vi "test_DMA Channels Input.vi"(8 "error in (no error)":errorcluster, 11 "TestCase in":refnum<class "DMA Channel Testing.lvclass">) -> (0 "error out":errorcluster, 3 "TestCase out":refnum<class "DMA Channel Testing.lvclass">)   [LabVIEW 2019, in "DMA Channel Testing.lvclass"]
uses:
  DMA Channel Testing.lvclass
  Addon/Addon Shared/Types/DMA Settings.ctl
  Addon/Addon Shared/Types/Delacing Scheme.ctl
  Addon/Addon Shared/Types/DMA Acquisition Mode.ctl
  DMA Channel Testing.lvclass/DMA Channel Testing.ctl
  Addon/Addon Shared/SubVIs/Constants.vi
  <vilib>/NI/NI VeriStand Advanced SysDef API/_SubVIs/SysDef.Search.GUID.vi
  <vilib>/NI/NI VeriStand Advanced SysDef API/_SubVIs/SysDef.Search.GUIDs.vi
  <vilib>/addons/_JKI Toolkits/VI Tester/TestCase.llb/TestCase.lvclass
  Addon/Addon System Explorer/FPGA Addon System Explorer.lvlib
  Addon/Addon Shared/FPGA Addon Shared.lvlib
  <vilib>/NI/NI VeriStand Advanced SysDef API/SysDef API/Advanced System Definition.lvlib
  C:/Program Files (x86)/National Instruments/LabVIEW 2019/vi.lib/addons/_JKI Toolkits/VI Tester/TestCase.llb/TestCase.lvclass
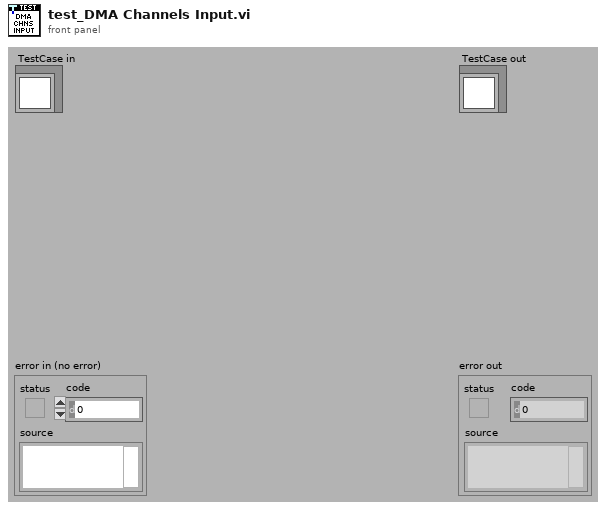
[diagram p1: front panel]
types:
  T1 = typedef "FPGA Addon Shared.lvlib/DMA Settings.ctl" = cluster{"Number of Channels":u8, "Delacing Scheme":T2, "Update Rate":u32, "dt":dbl, "Mode":T3, "Number of Samples":u32, "DMA Host Buffer":u32}
  T2 = typedef "FPGA Addon Shared.lvlib/Delacing Scheme.ctl" = enum8{"Interleaved", "Bitpacked"}
  T3 = typedef "FPGA Addon Shared.lvlib/DMA Acquisition Mode.ctl" = enum8{"Continuous", "Triggered Finite"}
  T4 = typedef "Advanced System Definition.lvlib/TreeItem.Info.ctl" = cluster{"Name":string, "Description":string, "GUID":string, "Is Channel":bool, "Channel":T5, "Is Waveform":bool, "Waveform":T7}
  T5 = typedef "Custom Device API.lvlib/Custom Device Channel.ctl" = cluster{"Type":T6, "Units":string, "Default Value":dbl, "Faultable":bool, "Scalable":bool}
  T6 = typedef "Custom Device API.lvlib/Custom Device Channel Type.ctl" = enum16{"Input", "Output"}
  T7 = typedef "Custom Device API.lvlib/Custom Device Waveform.ctl" = cluster{"Data Type":T8, "Units":string}
  T8 = typedef "Custom Device API.lvlib/Custom Device Waveform DataType.ctl" = enum16{"Double", "Complex Double"}
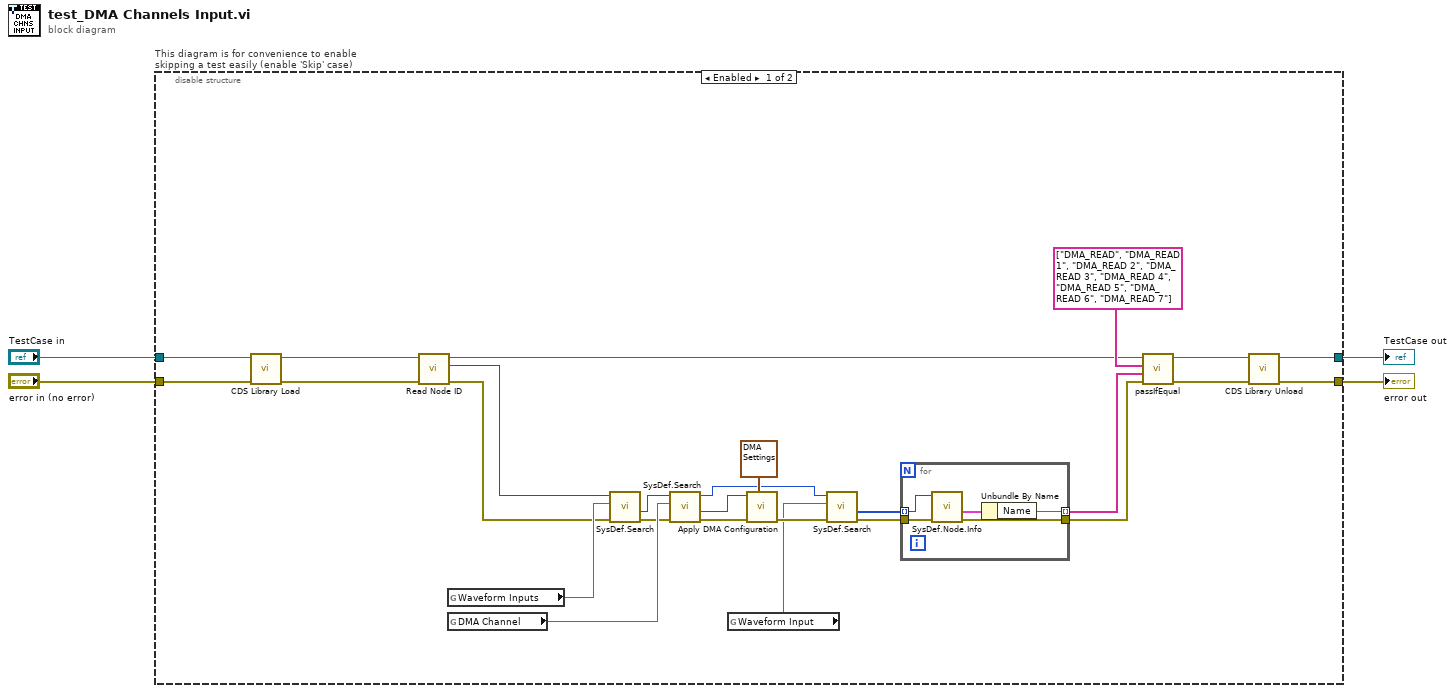
[diagram p0: block diagram]
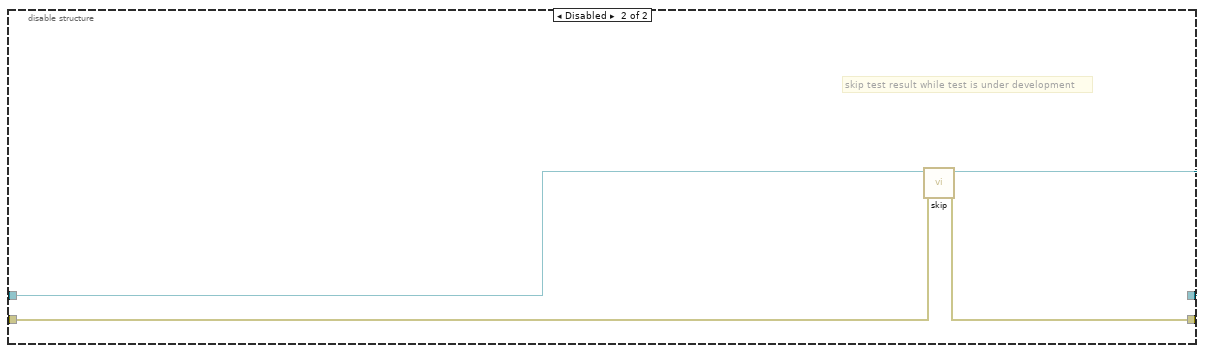
[diagram p2: hidden frame]
diagram:
  n1 = disable-structure "This diagram is for convenience to enable skipping a test easily (enable 'Skip' case)" shown="Enabled" {
    disable-tunnel: "TestCase in" -> [w11 w39]
    disable-tunnel: [w5 w37] -> w1
    disable-tunnel: [w6 w38] -> w3
    disable-tunnel: "error in (no error)" -> [w12 w36]
    frame Enabled {
      n2 = call "CDS Library Load.vi"("error in (no error)"=w12, "DMA Channel Testing in"=w11) -> ("error out"=w9:errorcluster, "DMA Channel Testing out"=w10:refnum<class "DMA Channel Testing.lvclass">)  [unwired: 8 in]
      n3 = call "Read Node ID.vi"("error in (no error)"=w9, "DMA Channel Testing in"=w10) -> ("error out"=w15:errorcluster, "Node ID"=w14:u64, "DMA Channel Testing out"=w13:refnum<class "DMA Channel Testing.lvclass">)  [unwired: 7 in]
      n4 = global read "Constants.vi" "Waveform Inputs"() -> (w28:string)
      n5 = global read "Constants.vi" "DMA Channel"() -> (w27:string)
      n6 = call-poly <vilib>:"SysDef.Search.vi"("error in (no error)"=w15, "GUID"=w28, "nodeID"=w14) -> ("error out"=w25:errorcluster, "Value out"=w26:u64)  [unwired: 5 in, 2 out]
      n7 = call-poly <vilib>:"SysDef.Search.vi"("error in (no error)"=w25, "GUID"=w27, "nodeID"=w26) -> ("error out"=w29:errorcluster, "Value out"=w24:u64, "nodeID out"=w21:u64)  [unwired: 5 in, 1 out]
      n8 = global read "Constants.vi" "Waveform Input"() -> (w22:string)
      n9 = call "Apply DMA Configuration.vi"("DMA Settings"=T1 {"Number of Channels"=8, "Delacing Scheme"=enum."Interleaved", "Update Rate"=0, "dt"=0.0, "Mode"=enum."Continuous", "Number of Samples"=0, "DMA Host Buffer"=0}, "error in (no error)"=w29, "Item Ref in"=w24) -> ("error out"=w23:errorcluster)  [unwired: 8 in]
      n10 = call-poly <vilib>:"SysDef.Search.vi"("error in (no error)"=w23, "GUID"=w22, "nodeID"=w21) -> ("error out"=w19:errorcluster, "Values Out"=w20:u64[])  [unwired: 5 in, 2 out]
      n11 = for {
        tunnel: w20 -> [w35] mode=indexing
        tunnel: w19 -> [w34]
        tunnel: [w33] -> w18
        tunnel: [w31] -> w17 mode=indexing
        n12 = call <vilib>:"SysDef.Node.Info.vi"("error in (no error)"=w34, "nodeID"=w35) -> ("error out"=w33:errorcluster, "Item Info"=w32:T4)  [unwired: 6 in, 2 out]
        n13 = Unbundle By Name(w32) -> ("Name"=w31:string)
      }
      n14 = call-dynamic "passIfEqual.vi"("error in (no error)"=w18, "y"=w17, "x"=string[] ["DMA_READ", "DMA_READ 1", "DMA_READ 2", "DMA_READ 3", "DMA_READ 4", "DMA_READ 5", "DMA_READ 6", "DMA_READ 7"] ("Array"), "TestCase in"=w13) -> ("error out"=w8:errorcluster, "TestCase out"=w7:refnum<class "DMA Channel Testing.lvclass">)  [unwired: 6 in]
      n15 = call "CDS Library Unload.vi"("error in (no error)"=w8, "DMA Channel Testing in"=w7) -> ("error out"=w6:errorcluster, "DMA Channel Testing out"=w5:refnum<class "DMA Channel Testing.lvclass">)  [unwired: 8 in]
    }
    frame Disabled {
      # "skip test result while test is under development"
      n16 = call <vilib>:"skip.vi"("error in (no error)"=w36, "TestCase in"=w39) -> ("error out"=w38:errorcluster, "TestCase out"=w37:refnum<class "DMA Channel Testing.lvclass">)  [unwired: 8 in]
    }
  }
  "error out" <- w3
  "TestCase out" <- w1
